vi "34330 Shunt Measurement.vi"(8 "error in (no error)":errorcluster, 11 "Volts Reading In":dbl) -> (0 "error out":errorcluster, 3 "Current Reading Out":string)   [LabVIEW 2015]
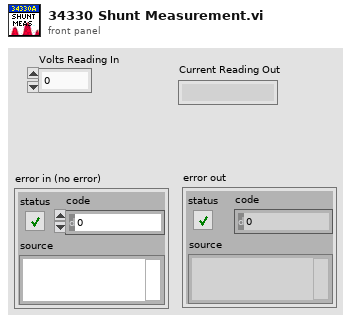
[diagram p1: front panel]
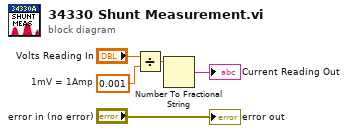
[diagram p0: block diagram]
diagram:
  w3 = 0.001  # 1mV = 1Amp
  n1 = Divide(x="Volts Reading In", y=w3) -> (x/y=w2:dbl)
  n2 = Number To Fractional String(number=w2) -> (F-format string=→"Current Reading Out":string)  [unwired: 3 in]
  "error out" <- "error in (no error)"
